vi "数据库清空对话框.vi"() -> ()   [LabVIEW 2016, in "数据查询.lvlib"]
panel:
  in  "布尔":bool
  in  "table":i32[](listbox)
  in  "database":enum16{"database1", "database3"}(ring)
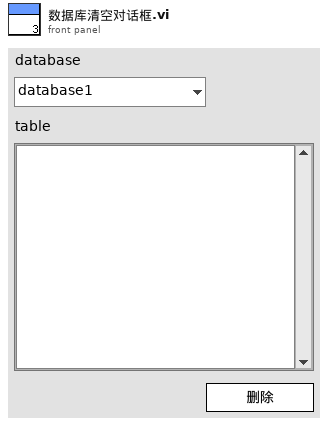
[diagram p1: front panel]
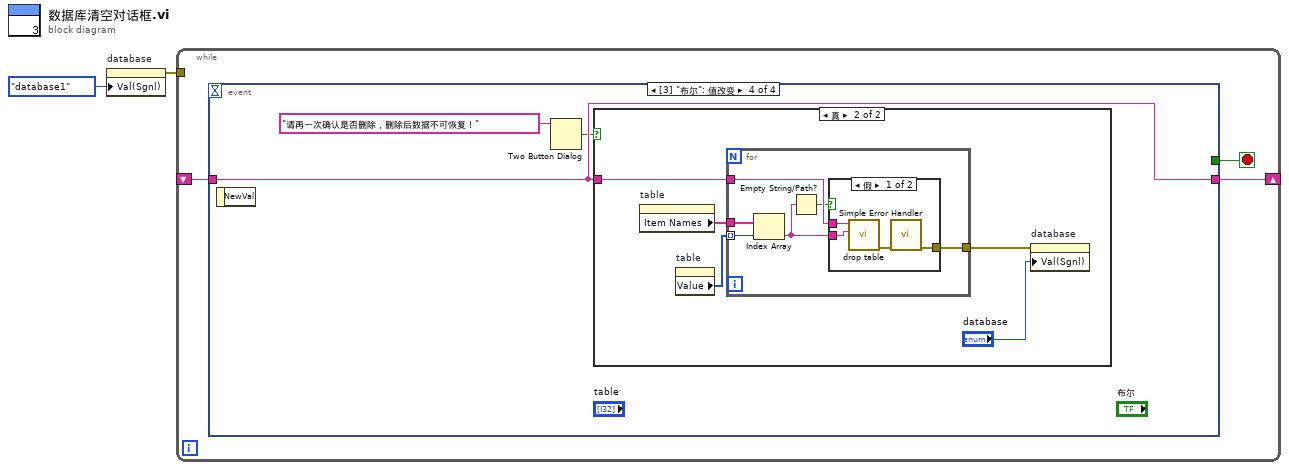
[diagram p0: block diagram]
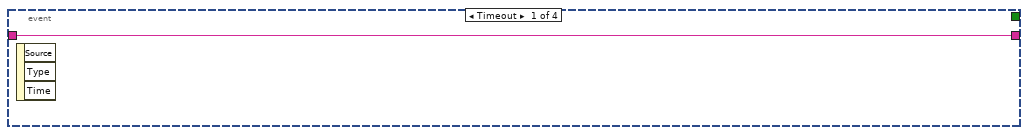
[diagram p2: hidden frame]
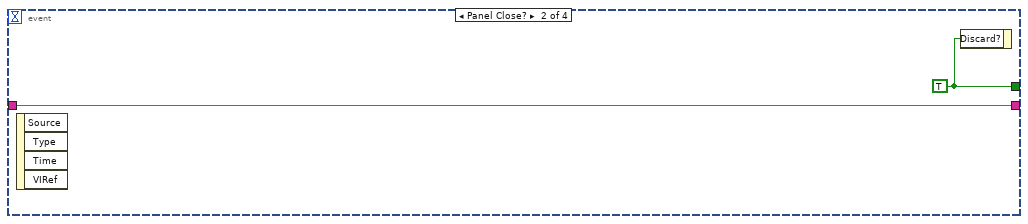
[diagram p3: hidden frame]
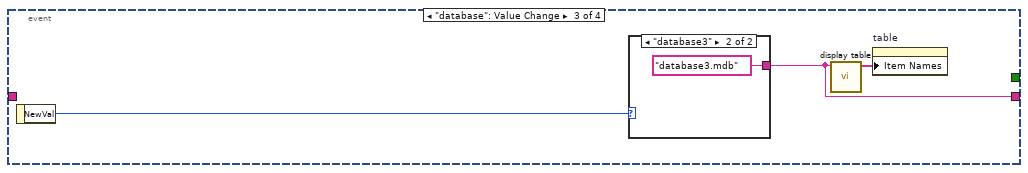
[diagram p4: hidden frame]
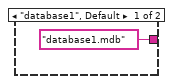
[diagram p5: hidden frame]
diagram:
  n1 = property on="database" class="Enum (严格)"("Val(Sgnl)"=enum16{"database1", "database3"}."database1" ("值(信号)")) -> (error out=w2:errorcluster)  [unwired: 2 in, 1 out]
  n2 = while {
    tunnel: w2 -> [_]
    shift-right: [w4] -> _
    shift-left: _ -> [w3]
    stop <- w5 stop-if-true
    n3 = event shown="[3] \"布尔\": 值改变" {
      selector: _ -> [_ _ _ _]
      dyn-events: _ -> [_ _ _ _]
      timeout: _ -> [_ _ _ _]
      tunnel: [_ w8 _ _] -> w5
      tunnel: [w6 w7 w9 w16] -> w4
      tunnel: w3 -> [w6 w7 _ w16]
      event Timeout {
        n4 = event-data() -> ()  [unwired: 1 in, 3 out]
      }
      event Panel Close? {
        w8 = TRUE
        n5 = event-data() -> ()  [unwired: 1 in, 4 out]
        n6 = event-data("Discard?"=w8) -> ()  [unwired: 1 in, 1 out]
      }
      event "database": Value Change {
        n7 = event-data() -> ("NewVal"=w11:enum16{"database1", "database3"})  [unwired: 1 in]
        n8 = case shown="\"database3\"" w11 {
          tunnel: ["database1.mdb" ("database") "database3.mdb" ("database")] -> w9
          frame "database1", Default {
          }
          frame "database3" {
          }
        }
        n9 = call "display table.vi"("database"=w9) -> ("tables"=w10:string[])  [unwired: 9 in, 1 out]
        n10 = property on="table" class="LstBox (严格)"("Item Names"=w10) -> ()  [unwired: 2 in, 2 out]
      }
      event "布尔": Value Change {
        n11 = event-data() -> ()  [unwired: 1 in, 1 out]
        n12 = Two Button Dialog(message="请再一次确认是否删除，删除后数据不可恢复！" ("消息")) -> (T button?=w15:bool)  [unwired: 2 in]
        n13 = case shown="真" w15 {
          tunnel: w16 -> [_ w19]
          frame False {
          }
          frame True {
            n14 = property on="table" class="LstBox (严格)"() -> ("Item Names"=w21:string[])  [unwired: 2 in, 2 out]
            n15 = property on="table" class="LstBox (严格)"() -> ("Value"=w20:i32[])  [unwired: 2 in, 2 out]
            n16 = for {
              tunnel: w21 -> [w27]
              tunnel: w20 -> [w26] mode=indexing
              tunnel: w19 -> [w25]
              tunnel: [w24] -> w17
              n17 = Index Array(array=w27, index=w26) -> (element=w23:string)
              n18 = Empty String/Path?(string/path=w23) -> (empty?=w22:bool)
              n19 = case shown="假" w22 {
                tunnel: w25 -> [w31 _]
                tunnel: [w29 _] -> w24
                tunnel: w23 -> [w28 _]
                frame False {
                  n20 = call "drop table.vi"("table"=w28, "database"=w31) -> ("error out"=w30:errorcluster)  [unwired: 9 in]
                  n21 = call <vilib>:"Simple Error Handler.vi"("error in (no error)"=w30) -> ("error out"=w29:errorcluster)  [unwired: 4 in, 4 out]
                }
                frame True {
                }
              }
            }
            n22 = property on="database" class="Enum (严格)"(error in=w17, "Val(Sgnl)"="database") -> ()  [unwired: 1 in, 2 out]
          }
        }
      }
    }
  }
